vi "OperateOnDigitalOutput.vi"(2 "error in (no error)":errorcluster, 3 "Image Settings":T1={"Start Position (µm)"={"x"=0.0, "y"=0.0, "z"=0.0}, "End Position (µm)"={"x"=10.0, "y"=10.0, "z"=0.0}, "Image Resolution (nm/pixel)"={"x"=50.0, "y"=50.0, "z"=100.0}, "Image Size (µm)"={"x"=10.0, "y"=10.0, "z"=0.0}, "Image Size (pixel)"={"x"=50, "y"=50, "z"=0}, "Time Resolution\n(ms/pixel)"=7.0, "1st Axis"=0, "2nd Axis"=1, "Retrace"=FALSE, "Estimated Time"=""} {"2nd Axis" items=["x", "y", "z"]; "1st Axis" items=["x", "y", "z"]; "Time Resolution\n(ms/pixel)" format="%.2f"; "Image Resolution (nm/pixel)"."z" format="%.2f"; "Image Resolution (nm/pixel)"."y" format="%.2f"; "Image Resolution (nm/pixel)"."x" format="%.2f"; "Image Size (µm)"."z" format="%.2f"; "Image Size (µm)"."y" format="%.2f"; "Image Size (µm)"."x" format="%.2f"; "End Position (µm)"."z" format="%.2f"; "End Position (µm)"."y" format="%.2f"; "End Position (µm)"."x" format="%.2f"; "Start Position (µm)"."z" format="%.2f"; "Start Position (µm)"."y" format="%.2f"; "Start Position (µm)"."x" format="%.2f"}, 4 "operation":enum16{"start", "state", "abort"}(ring)) -> (0 "error out":errorcluster)   [LabVIEW 2009]
uses:
  ImageSettings.ctt
panel:
  out "Position":dbl[](array[numeric]) format="%.6f"
  out "Velocity":dbl[](array[numeric]) format="%.6f"
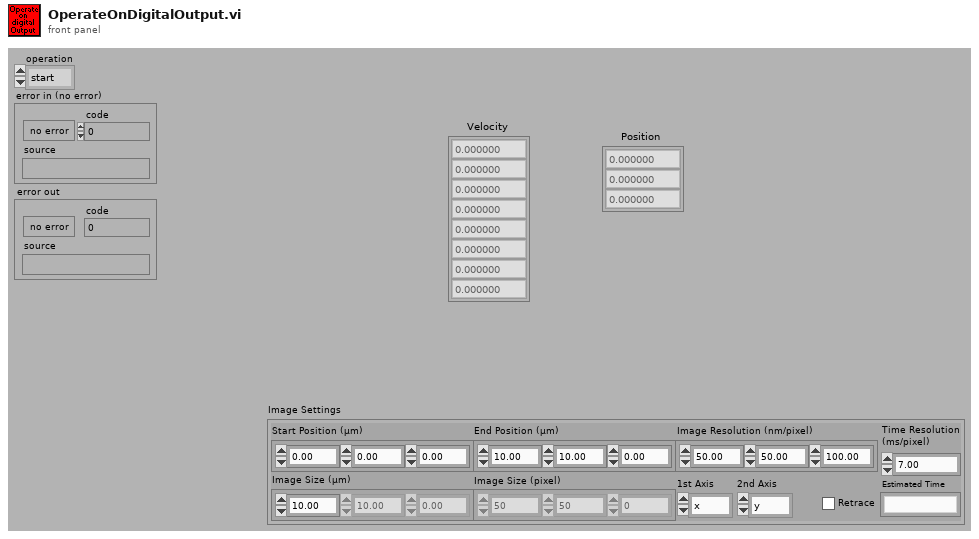
[diagram p1: front panel]
types:
  T1 = typedef "ImageSettings.ctt" = cluster{"Start Position (µm)":cluster{"x":dbl, "y":dbl, "z":dbl}, "End Position (µm)":cluster{"x":dbl, "y":dbl, "z":dbl}, "Image Resolution (nm/pixel)":cluster{"x":dbl, "y":dbl, "z":dbl}, "Image Size (µm)":cluster{"x":dbl, "y":dbl, "z":dbl}, "Image Size (pixel)":cluster{"x":u32, "y":u32, "z":u32}, "Time Resolution\n(ms/pixel)":dbl, "1st Axis":u16, "2nd Axis":u16, "Retrace":bool, "Estimated Time":string}
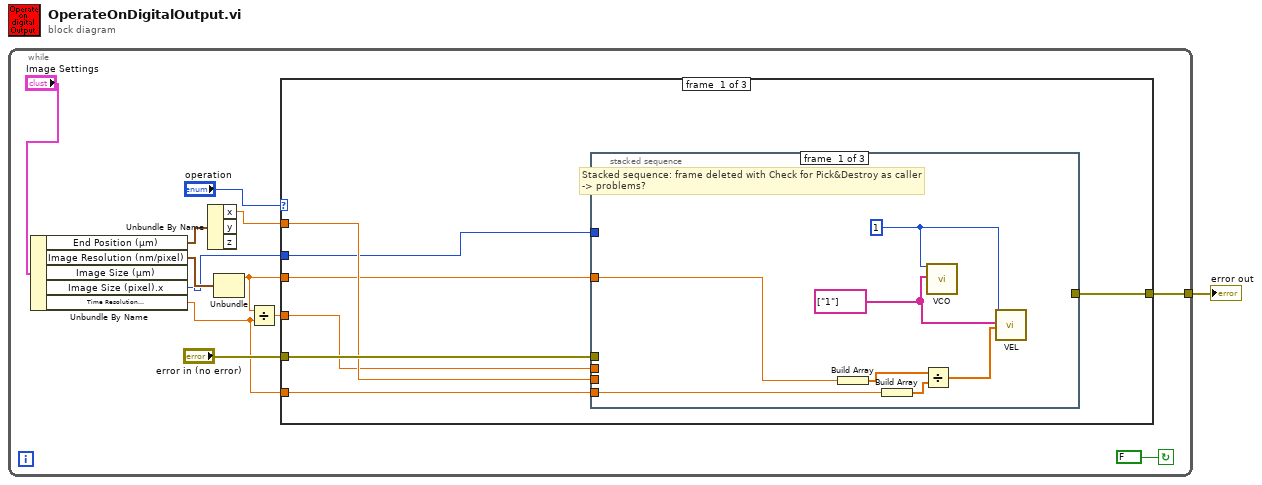
[diagram p0: block diagram]
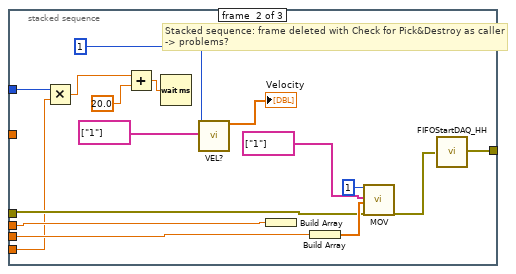
[diagram p2: hidden frame]
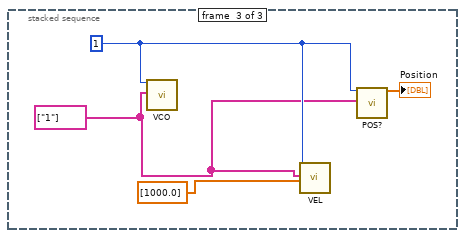
[diagram p3: hidden frame]
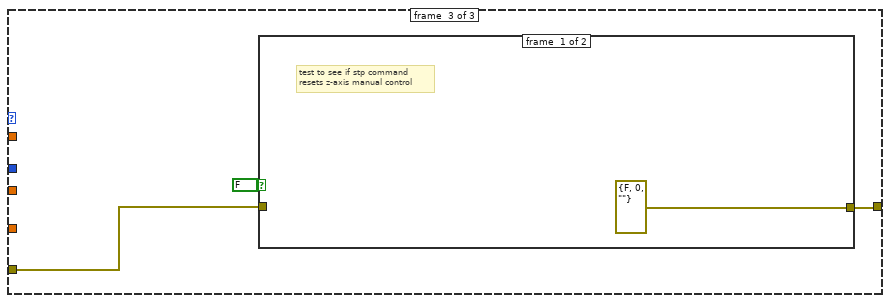
[diagram p5: hidden frame]
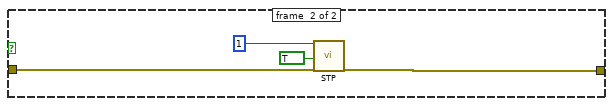
[diagram p6: hidden frame]
diagram:
  n1 = while {
    tunnel: [w10] -> w1
    stop <- FALSE continue-if-true
    n2 = Unbundle By Name("Image Settings") -> ("End Position (µm)"=w8:cluster{"x":dbl, "y":dbl, "z":dbl}, "Image Resolution (nm/pixel)"=w7:cluster{"x":dbl, "y":dbl, "z":dbl}, "Image Size (pixel).x"=w2:u32, "Time Resolution\n(ms/pixel)"=w3:dbl)  [unwired: 1 out]
    n3 = Unbundle By Name(w8) -> ("x"=w6:dbl)  [unwired: 2 out]
    n4 = Unbundle(w7) -> ("x"=w4:dbl)  [unwired: 2 out]
    n5 = Divide(x=w4, y=w3) -> (x/y=w5:dbl)
    n6 = case shown="\"start\", Default" "operation" {
      tunnel: "error in (no error)" -> [w19 w48 w51]
      tunnel: [w20 w48 w50] -> w10
      tunnel: w6 -> [w18 _ _]
      tunnel: w5 -> [w17 _ _]
      tunnel: w4 -> [w16 _ _]
      tunnel: w3 -> [w15 _ _]
      tunnel: w2 -> [w14 _ _]
      frame #0 {
        n7 = stacked-sequence {
          tunnel: [_ w43 _] -> w20
          tunnel: w19 -> [_ w39 _]
          tunnel: w18 -> [_ w42 _]
          tunnel: w17 -> [_ w40 _]
          tunnel: w16 -> [w27 _ _]
          tunnel: w15 -> [w26 w32 _]
          tunnel: w14 -> [_ w29 _]
          frame #0 {
            w21 = string[] ["1"] ("Axes to move")
            w22 = 1 ("System no.")
            # "Stacked sequence: frame deleted with Check for Pick&Destroy as caller\n-> problems?"
            n8 = Build Array(w27) -> (w25:dbl[])
            n9 = Build Array(w26) -> (w24:dbl[])
            n10 = Divide(x=w25, y=w24) -> (x/y=w23:dbl[])
            n11 = call "VCO.vi"("System no."=w22, "Axes to command"=w21) -> ()  [unwired: 17 in, 1 out]
            n12 = call "VEL.vi"("System no."=w22, "Axes to set"=w21, "Velocity values"=w23) -> ()  [unwired: 15 in, 2 out]
          }
          frame #1 {
            # "Stacked sequence: frame deleted with Check for Pick&Destroy as caller\n-> problems?"
            n13 = Multiply(x=w29, y=w32) -> (x*y=w30:dbl)
            n14 = Add(x=w30, y=20.0) -> (x+y=w28:dbl)
            n15 = Wait (ms)(milliseconds to wait=w28) -> ()  [unwired: 1 out]
            n16 = call "VEL?.vi"("System no."=1, "Axes to query"=string[] ["1"] ("Axes to move")) -> ("Velocity"=→"Velocity":dbl[])  [unwired: 16 in, 1 out]
            n17 = Build Array(w40) -> ()  [unwired: 1 out]
            n18 = Build Array(w42) -> (w41:dbl[])
            n19 = call "MOV.vi"("System no."=1, "Axes to move"=string[] ["1"], "Position values"=w41, "error in"=w39) -> ("error out"=w35:errorcluster)  [unwired: 15 in]
            n20 = call "FIFOStartDAQ_HH.vi"("error in (no error)"=w35) -> ("error out"=w43:errorcluster)
          }
          frame #2 {
            w44 = string[] ["1"] ("Axes to move")
            w47 = 1 ("System no.")
            n21 = call "VCO.vi"("System no."=w47, "Axes to command"=w44) -> ()  [unwired: 17 in, 1 out]
            n22 = call "VEL.vi"("System no."=w47, "Axes to set"=w44, "Velocity values"=dbl[] [1000.0]) -> ()  [unwired: 15 in, 2 out]
            n23 = call "POS?.vi"("System no."=w47, "Axes to query"=w44) -> ("Position"=→"Position":dbl[])  [unwired: 16 in, 1 out]
          }
        }
      }
      frame #1 {
      }
      frame #2 {
        n24 = case shown="False" FALSE {
          tunnel: w51 -> [_ w56]
          tunnel: [errorcluster {"status"=FALSE, "code"=0, "source"=""} ("error out") w53] -> w50
          frame #0 {
            # "test to see if stp command\nresets z-axis manual control"
          }
          frame #1 {
            n25 = call "STP.vi"("System no."=1, "All axes?"=TRUE, "error in"=w56) -> ("error out"=w53:errorcluster)  [unwired: 16 in]
          }
        }
      }
    }
  }
  "error out" <- w1
